vi "GetAllEnqueue.vi"(8 "error in (no error)":errorcluster, 11 "ActorMap in":refnum<class "ActorMap.lvclass">) -> (0 "error out":errorcluster, 1 "Names":string[](array[string]), 2 "Enqueues":refnum<class "Message Enqueuer.lvclass">[](array[class]), 3 "ActorMap out":refnum<class "ActorMap.lvclass">)   [LabVIEW 2020, in "ActorMap.lvclass"]
uses:
  ActorMap.lvclass
  <vilib>/ActorFramework/Message Enqueuer/Message Enqueuer.lvclass
  ActorMap.lvclass/ActorMap.ctl
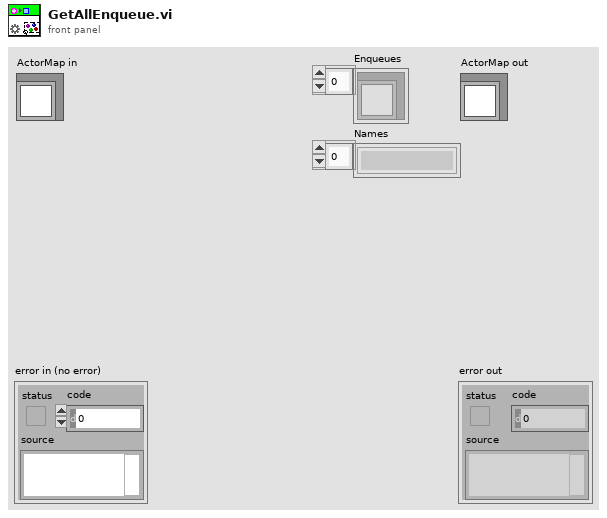
[diagram p1: front panel]
types:
  T1 = map{string, refnum<class "Message Enqueuer.lvclass">}
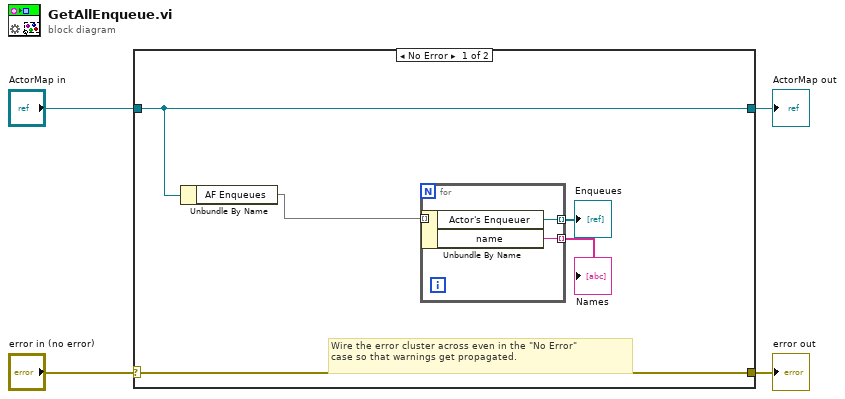
[diagram p0: block diagram]
diagram:
  n1 = case shown="No Error" "error in (no error)" {
    selector: "error in (no error)" -> [w9 w14]
    tunnel: [w9 w14] -> w3
    tunnel: [w8 w13] -> w1
    tunnel: "ActorMap in" -> [w8 w13]
    frame No Error {
      # "Wire the error cluster across even in the \"No Error\"\ncase so that warnings get propagated."
      n2 = Unbundle By Name(w8) -> ("AF Enqueues"=w7:T1)
      n3 = for {
        tunnel: w7 -> [w12] mode=indexing
        tunnel: [w11] -> w6 mode=indexing
        tunnel: [w10] -> w5 mode=indexing
        n4 = Unbundle By Name(w12) -> ("Actor's Enqueuer"=w11:refnum<class "Message Enqueuer.lvclass">, "name"=w10:string)
      }
      "Enqueues" <- w6
      "Names" <- w5
    }
    frame Error {
    }
  }
  "error out" <- w3
  "ActorMap out" <- w1
